vi "Setup.vi"(8 "error in (no error)":errorcluster, 11 "LUnit Test Max File Size (SQL) In":refnum<class "Test Max File Size (SQL).lvclass">) -> (0 "error out":errorcluster, 3 "LUnit Test Max File Size (SQL) Out":refnum<class "Test Max File Size (SQL).lvclass">)   [LabVIEW 2019, in "Test Max File Size (SQL).lvclass"]
doc: "Setup method called by the testing framework to set up test fixture before each test method is called."
uses:
  Test Max File Size (SQL).lvclass
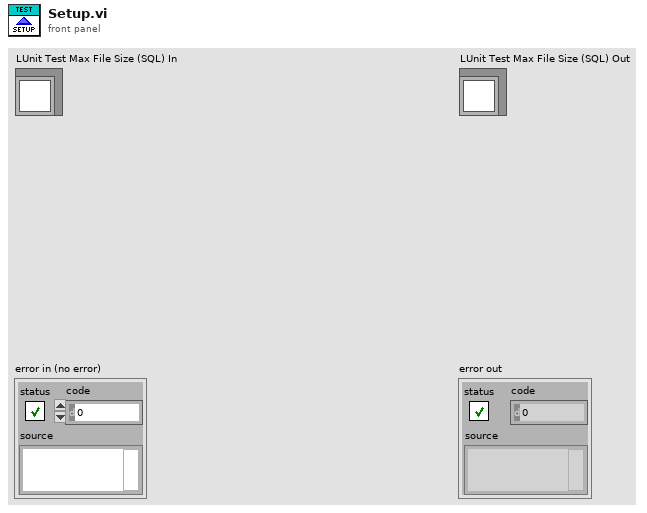
[diagram p1: front panel]
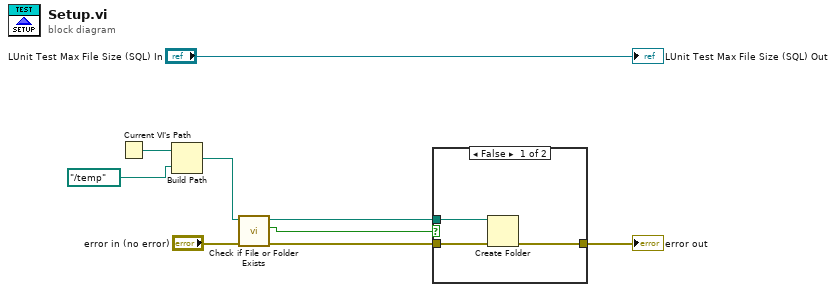
[diagram p0: block diagram]
diagram:
  n1 = Current VI's Path() -> (path=w8:path)
  n2 = Build Path(base path=w8, name or relative path=path "../temp") -> (appended path=w5:path)
  n3 = call <vilib>:"Check if File or Folder Exists.vi"("error in (no error)"="error in (no error)", "path"=w5) -> ("error out"=w6:errorcluster, "file or folder exists?"=w3:bool, "dup path"=w4:path)  [unwired: 7 in]
  n4 = case shown="False" w3 {
    tunnel: w6 -> [w12 w13]
    tunnel: [w11 w13] -> w1
    tunnel: w4 -> [w10 _]
    frame False {
      n5 = Create Folder(path (use dialog)=w10, error in=w12) -> (error out=w11:errorcluster)  [unwired: 1 in, 2 out]
    }
    frame True {
    }
  }
  "error out" <- w1
  "LUnit Test Max File Size (SQL) Out" <- "LUnit Test Max File Size (SQL) In"
